vi "Obtain Queue.vi"(8 "error in (no error)":errorcluster, 9 "Max Queue Size":u32=2, 10 "# of Priorities":i32=2) -> (0 "error out":errorcluster, 3 "Bounded Priority Queue":refnum<class "Bounded Priority Queue.lvclass">)   [LabVIEW 2011, in "Bounded Priority Queue.lvclass"]
uses:
  Bounded Priority Queue.lvclass
  DVR Contents.ctl
  Data.ctl
  Bounded Priority Queue.lvclass/Bounded Priority Queue.ctl
panel:
  in  "Illegal size":string="Illegal maximum queue size. Queue size must be negative for unlimited or 2 or greater.  Values of zero or one make no sense for a priority queue. If you want a single element queue, use a non-priority queue."
  in  "# of Priorities must be positive":string="# of Priorities input must be a positive number, not zero or negative."
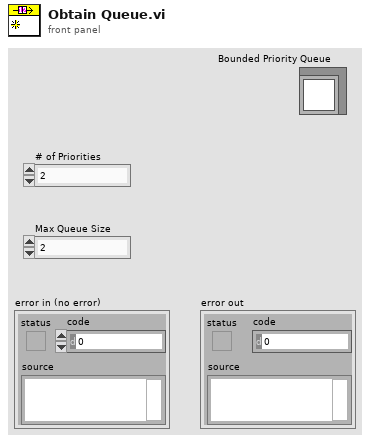
[diagram p1: front panel]
types:
  T1 = typedef "Bounded Priority Queue.lvclass/DVR Contents.ctl" = cluster{"# Waiting":u32, "Buffers":refnum<queue>[], "How Many Priorities":u32, "Bounding":refnum<queue>}
  T2 = typedef "Bounded Priority Queue.lvclass/Data.ctl" = string
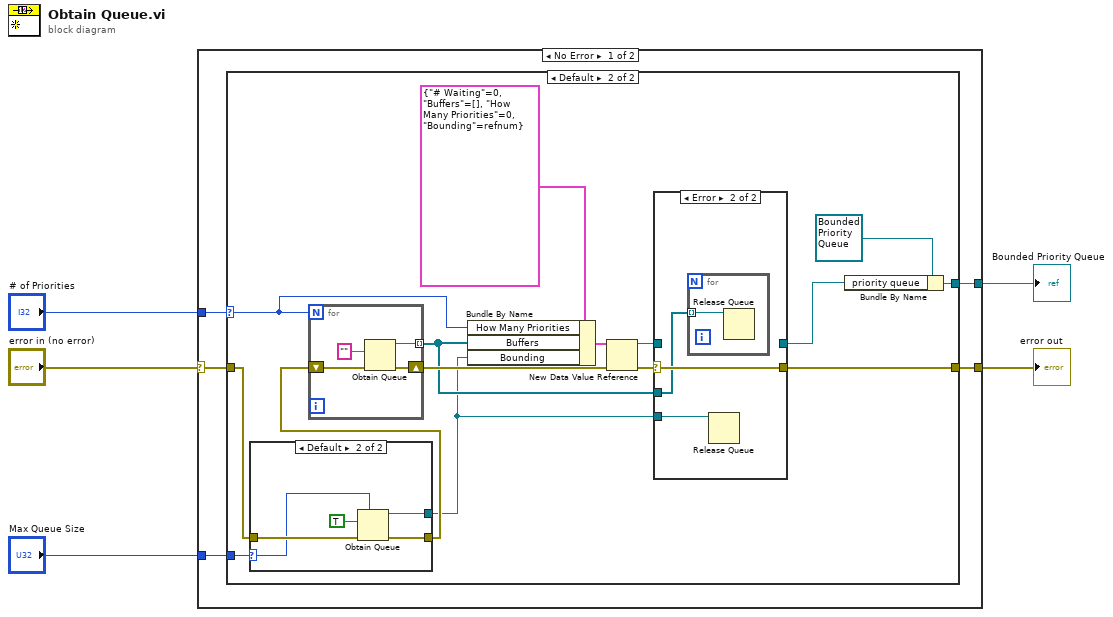
[diagram p0: block diagram]
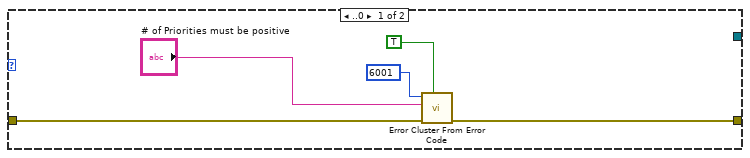
[diagram p2: hidden frame]
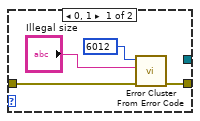
[diagram p3: hidden frame]
diagram:
  n1 = case shown="No Error" "error in (no error)" {
    selector: "error in (no error)" -> [w7 w50]
    tunnel: [w10 w50] -> w5
    tunnel: [w9 _] -> w4
    tunnel: "# of Priorities" -> [w8 _]
    tunnel: "Max Queue Size" -> [w6 _]
    frame No Error {
      n2 = case shown="Default" w8 {
        selector: w8 -> [_ w20]
        tunnel: [w12 w27] -> w10
        tunnel: [_ w21] -> w9
        tunnel: w7 -> [w11 w18]
        tunnel: w6 -> [_ w19]
        frame ..0 {
          n3 = call <vilib>:"Error Cluster From Error Code.vi"("show call chain? (False)"=TRUE, "error in (no error)"=w11, "error message (\"\")"="# of Priorities must be positive", "error code (0)"=6001) -> ("error out"=w12:errorcluster)  [unwired: 5 in]
        }
        frame Default {
          n4 = case shown="Default" w19 {
            selector: w19 -> [_ w36]
            tunnel: w18 -> [w32 w39]
            tunnel: [w31 w38] -> w17
            tunnel: [_ w35] -> w16
            frame 0, 1 {
              n5 = call <vilib>:"Error Cluster From Error Code.vi"("error in (no error)"=w32, "error message (\"\")"="Illegal size", "error code (0)"=6012) -> ("error out"=w31:errorcluster)  [unwired: 6 in]
            }
            frame Default {
              n6 = Obtain Queue(max queue size (-1, unlimited)=w36, element data type=TRUE, error in (no error)=w39) -> (queue out=w35:refnum<queue>, error out=w38:errorcluster)  [unwired: 2 in, 1 out]
            }
          }
          n7 = for {
            N: w20 -> [_]
            tunnel: [w48] -> w25 mode=indexing
            shift-right: [w47] -> w30
            shift-left: w17 -> [w46]
            n8 = Obtain Queue(element data type=T2 "" ("Data"), error in (no error)=w46) -> (queue out=w48:refnum<queue>, error out=w47:errorcluster)  [unwired: 3 in, 1 out]
          }
          n9 = Bundle By Name(cluster=T1 {"# Waiting"=0, "Buffers"=[], "How Many Priorities"=0, "Bounding"=refnum} ("Priority Queue Internals"), "How Many Priorities"=w20, "Buffers"=w25, "Bounding"=w16) -> (w26:T1)
          n10 = New Data Value Reference(data value=w26, error in=w30) -> (data value reference=w28:refnum<data-value>, error out=w29:errorcluster)
          n11 = case shown="Error" w29 {
            selector: w29 -> [w40 w44]
            tunnel: w28 -> [w41 _]
            tunnel: [w41 _] -> w23
            tunnel: [w40 w44] -> w27
            tunnel: w25 -> [_ w43]
            tunnel: w16 -> [_ w42]
            frame No Error {
            }
            frame Error {
              n12 = for {
                tunnel: w43 -> [w45] mode=indexing
                n13 = Release Queue(queue=w45) -> ()  [unwired: 2 in, 3 out]
              }
              n14 = Release Queue(queue=w42) -> ()  [unwired: 2 in, 3 out]
            }
          }
          n15 = Bundle By Name(cluster=refnum<class "Bounded Priority Queue.lvclass"> refnum ("Priority Queue.lvclass"), "priority queue"=w23) -> (w21:refnum<class "Bounded Priority Queue.lvclass">)
        }
      }
    }
    frame Error {
    }
  }
  "error out" <- w5
  "Bounded Priority Queue" <- w4
